vi "Global 1.vi"() -> ()   [LabVIEW 2013]
panel:
  out "FER":dbl
  out "Синхр":bool
  out "Decode":bool[](array[boolean])
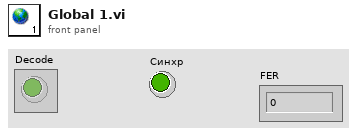
[diagram p1: front panel]
diagram:
